vi "Autonomous Independent.vi"() -> ()   [LabVIEW 2013]
doc: "This VI is called when autonomous begins, and will automatically be terminated when autonomous ends. You can carry out timed or sensor driven robot movement independently without needing to return to the caller."
uses:
  Robot Global Data.vi
  <vilib>/Rock Robotics/WPI/RobotDrive/WPI_RobotDriveGetSetRefNum.vi
  <vilib>/Rock Robotics/WPI/RobotDrive/WPI_RobotDriveArcadeDrive_Standard(NoSaturation).vi
  <vilib>/Rock Robotics/WPI/Joystick/WPI_JoystickGetSetRefNum.vi
panel:
  out "Current Movement, for debugging":T1 {"Y Joystick Value" scale=1.0..-1.0; "X Joystick Value" scale=-1.0..1.0}
  in  "Array of robot movements":T2(array[cluster])=[{"X Joystick Value"=0.0, "Y Joystick Value"=0.0, "Delay (sec)"=0.7, "Movement Name"="Lift Arm V", "Joystick Button 1"=FALSE, "Joystick Button 2"=TRUE, "Joystick Button 3"=FALSE, "Joystick Button 4"=FALSE, "Joystick Button 5"=FALSE, "Joystick Button 6"=FALSE, "Joystick Button 7"=FALSE, "Joystick Button 8"=FALSE, "Joystick Button 9"=FALSE, "Joystick Button 10"=FALSE, "Joystick Button 11"=FALSE, "Joystick Button 12"=FALSE}, {"X Joystick Value"=0.0, "Y Joystick Value"=0.0, "Delay (sec)"=0.5, "Movement Name"="Throw Arm V", "Joystick Button 1"=TRUE, "Joystick Button 2"=FALSE, "Joystick Button 3"=FALSE, "Joystick Button 4"=FALSE, "Joystick Button 5"=TRUE, "Joystick Button 6"=FALSE, "Joystick Button 7"=FALSE, "Joystick Button 8"=FALSE, "Joystick Button 9"=FALSE, "Joystick Button 10"=FALSE, "Joystick Button 11"=FALSE, "Joystick Button 12"=FALSE}, {"X Joystick Value"=-0.45, "Y Joystick Value"=-0.75, "Delay (sec)"=3.0, "Movement Name"="Drive Fwd", "Joystick Button 1"=FALSE, "Joystick Button 2"=FALSE, "Joystick Button 3"=FALSE, "Joystick Button 4"=FALSE, "Joystick Button 5"=FALSE, "Joystick Button 6"=FALSE, "Joystick Button 7"=FALSE, "Joystick Button 8"=FALSE, "Joystick Button 9"=FALSE, "Joystick Button 10"=FALSE, "Joystick Button 11"=FALSE, "Joystick Button 12"=FALSE}, {"X Joystick Value"=0.0, "Y Joystick Value"=0.0, "Delay (sec)"=0.5, "Movement Name"="Throw Arm ^", "Joystick Button 1"=TRUE, "Joystick Button 2"=FALSE, "Joystick Button 3"=FALSE, "Joystick Button 4"=FALSE, "Joystick Button 5"=TRUE, "Joystick Button 6"=FALSE, "Joystick Button 7"=FALSE, "Joystick Button 8"=FALSE, "Joystick Button 9"=FALSE, "Joystick Button 10"=FALSE, "Joystick Button 11"=FALSE, "Joystick Button 12"=FALSE}, {"X Joystick Value"=0.0, "Y Joystick Value"=0.0, "Delay (sec)"=1.0, "Movement Name"="Finish", "Joystick Button 1"=FALSE, "Joystick Button 2"=FALSE, "Joystick Button 3"=FALSE, "Joystick Button 4"=FALSE, "Joystick Button 5"=FALSE, "Joystick Button 6"=FALSE, "Joystick Button 7"=FALSE, "Joystick Button 8"=FALSE, "Joystick Button 9"=FALSE, "Joystick Button 10"=FALSE, "Joystick Button 11"=FALSE, "Joystick Button 12"=FALSE}, {"X Joystick Value"=0.0, "Y Joystick Value"=0.0, "Delay (sec)"=0.0, "Movement Name"="", "Joystick Button 1"=FALSE, "Joystick Button 2"=FALSE, "Joystick Button 3"=FALSE, "Joystick Button 4"=FALSE, "Joystick Button 5"=FALSE, "Joystick Button 6"=FALSE, "Joystick Button 7"=FALSE, "Joystick Button 8"=FALSE, "Joystick Button 9"=FALSE, "Joystick Button 10"=FALSE, "Joystick Button 11"=FALSE, "Joystick Button 12"=FALSE}, {"X Joystick Value"=0.0, "Y Joystick Value"=0.0, "Delay (sec)"=0.0, "Movement Name"="", "Joystick Button 1"=FALSE, "Joystick Button 2"=FALSE, "Joystick Button 3"=FALSE, "Joystick Button 4"=FALSE, "Joystick Button 5"=FALSE, "Joystick Button 6"=FALSE, "Joystick Button 7"=FALSE, "Joystick Button 8"=FALSE, "Joystick Button 9"=FALSE, "Joystick Button 10"=FALSE, "Joystick Button 11"=FALSE, "Joystick Button 12"=FALSE}, {"X Joystick Value"=0.0, "Y Joystick Value"=0.0, "Delay (sec)"=0.0, "Movement Name"="", "Joystick Button 1"=FALSE, "Joystick Button 2"=FALSE, "Joystick Button 3"=FALSE, "Joystick Button 4"=FALSE, "Joystick Button 5"=FALSE, "Joystick Button 6"=FALSE, "Joystick Button 7"=FALSE, "Joystick Button 8"=FALSE, "Joystick Button 9"=FALSE, "Joystick Button 10"=FALSE, "Joystick Button 11"=FALSE, "Joystick Button 12"=FALSE}] {"Y Joystick Value" scale=1.0..-1.0; "X Joystick Value" scale=-1.0..1.0}
  # "Be sure to right-click on the ARRAY object (not the individual elements) and choose Data Operations>>Make Current Value default if you want to save the array values with the VI"
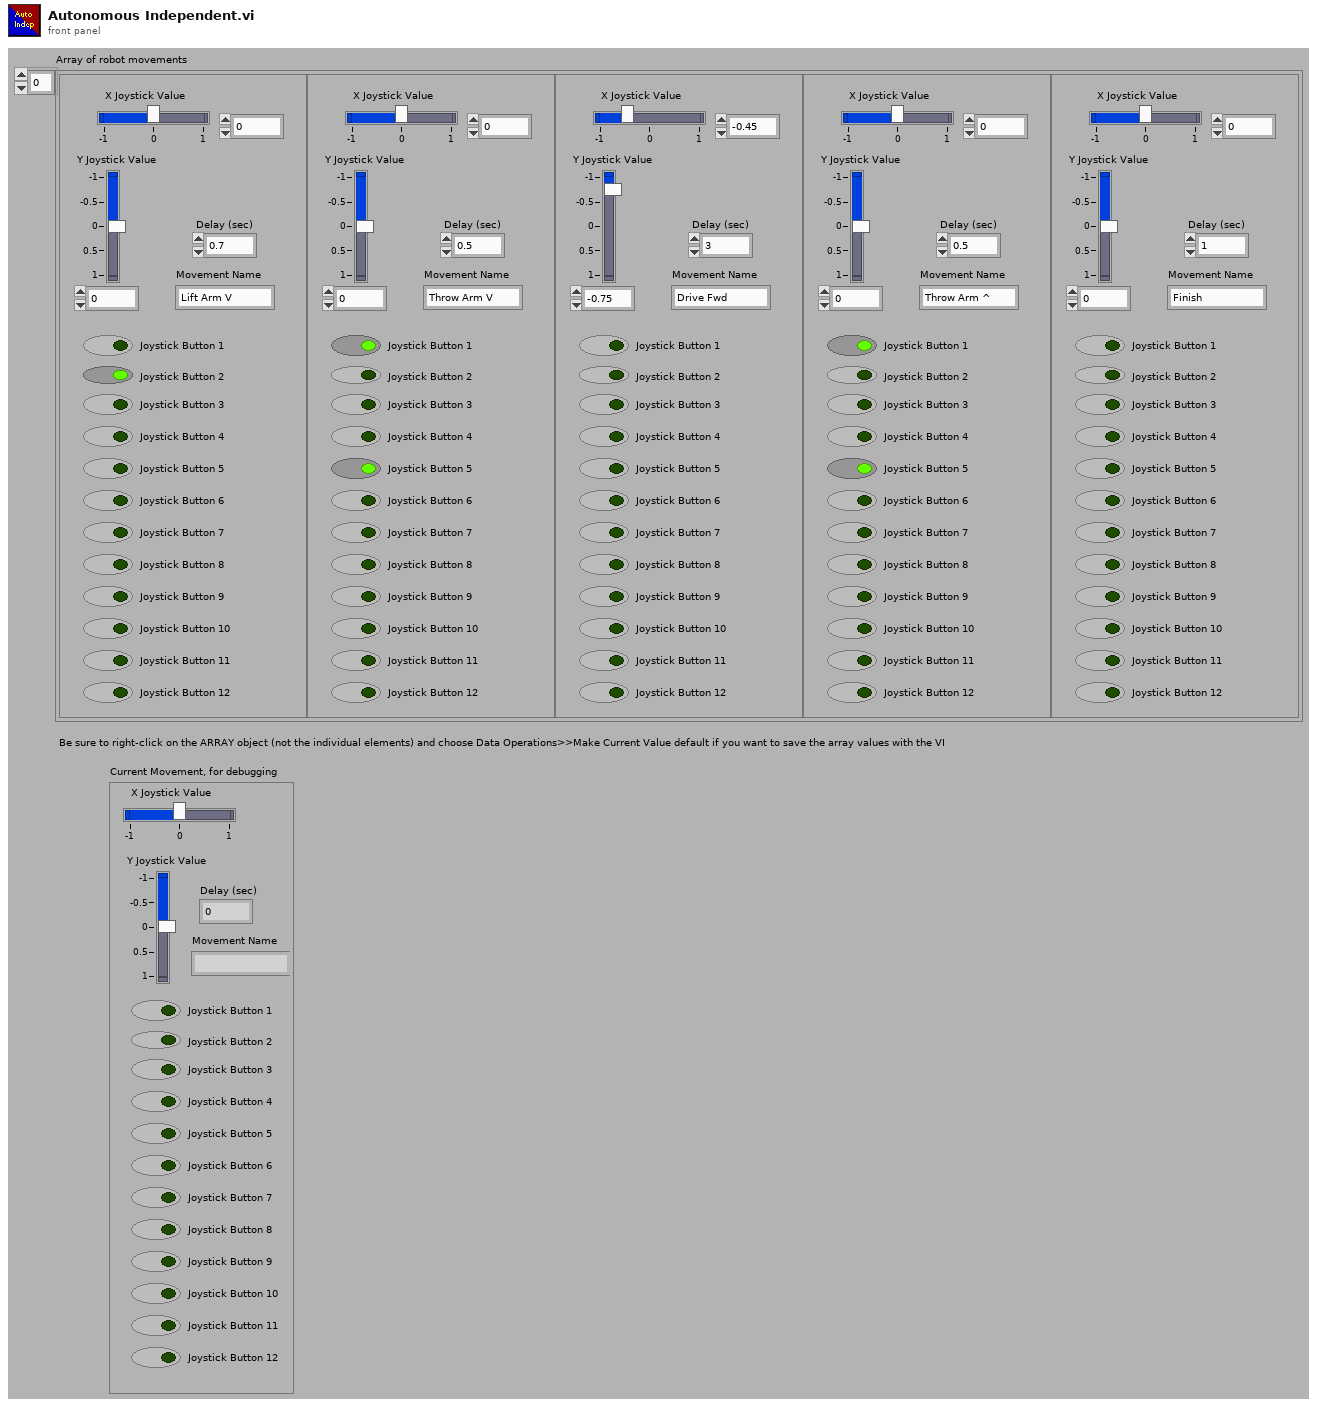
[diagram p1: front panel]
types:
  T1 = cluster{"X Joystick Value":dbl, "Y Joystick Value":dbl, "Delay (sec)":dbl, "Movement Name":string, "Joystick Button 1":bool, "Joystick Button 2":bool, "Joystick Button 3":bool, "Joystick Button 4":bool, "Joystick Button 5":bool, "Joystick Button 6":bool, "Joystick Button 7":bool, "Joystick Button 8":bool, "Joystick Button 9":bool, "Joystick Button 10":bool, "Joystick Button 11":bool, "Joystick Button 12":bool}
  T2 = cluster{"X Joystick Value":dbl, "Y Joystick Value":dbl, "Delay (sec)":dbl, "Movement Name":string, "Joystick Button 1":bool, "Joystick Button 2":bool, "Joystick Button 3":bool, "Joystick Button 4":bool, "Joystick Button 5":bool, "Joystick Button 6":bool, "Joystick Button 7":bool, "Joystick Button 8":bool, "Joystick Button 9":bool, "Joystick Button 10":bool, "Joystick Button 11":bool, "Joystick Button 12":bool}[]
  T3 = typedef "WPI_JoystickDevRef.ctl" = cluster{"Device":T4}
  T4 = typedef "WPI_JoystickDeviceEnum.ctl" = enum16{"USB 1", "USB 2", "USB 3", "USB 4", "Kinect 1", "Kinect 2"}
  T5 = cluster{"axis 1 (x)":dbl, "axis 2 (y)":dbl, "axis 3 (throttle)":dbl, "axis 4":dbl, "axis 5":dbl, "axis 6":dbl}
  T6 = typedef "WPI_RobotDriveDevRef.ctl" = cluster{"DevStatus":errorcluster, "Motors[]":T7[], "Square Inputs":bool, "Max Output":dbl, "Isochronous":bool}
  T7 = typedef "WPI_MotorControlDeviceRef.ctl" = cluster{"DeviceStatus":errorcluster, "Type":enum16{"PWM", "CAN"}, "PWM":cluster{"Digital Module":T8, "PWM Channel":T9, "DeadBand":T10}, "CAN":cluster{"Device Number":u8, "Control Mode":T11, "Semaphore":T12, "Max Vout":dbl}, "Invert":bool, "TransformRef":T13, "InvTransformRef":T13}
  T8 = typedef "FPGA_TypedefDigitalModule.ctl" = enum16{"Digital Module 1", "Digital Module 2"}
  T9 = typedef "FPGA_DIOPWMChannel.ctl" = enum8{"PWM 1", "PWM 2", "PWM 3", "PWM 4", "PWM 5", "PWM 6", "PWM 7", "PWM 8", "PWM 9", "PWM 10", "Invalid"}
  T10 = typedef "WPI_PWMDeadband.ctl" = cluster{"Name":string, "maxPositivePwm":i32, "minPositivePwm":i32, "centerPwm":i32, "maxNegativePwm":i32, "minNegativePwm":i32, "angularRange":u16}
  T11 = typedef "WPI_CANJaguar_ControlMode.ctl" = enum8{"Percent VBus", "Current", "Speed", "Position", "Voltage"}
  T12 = typedef "Semaphore RefNum" = refnum<k1>
  T13 = typedef "WPI_PWMTransform_ConPane.ctl" = refnum<vi>
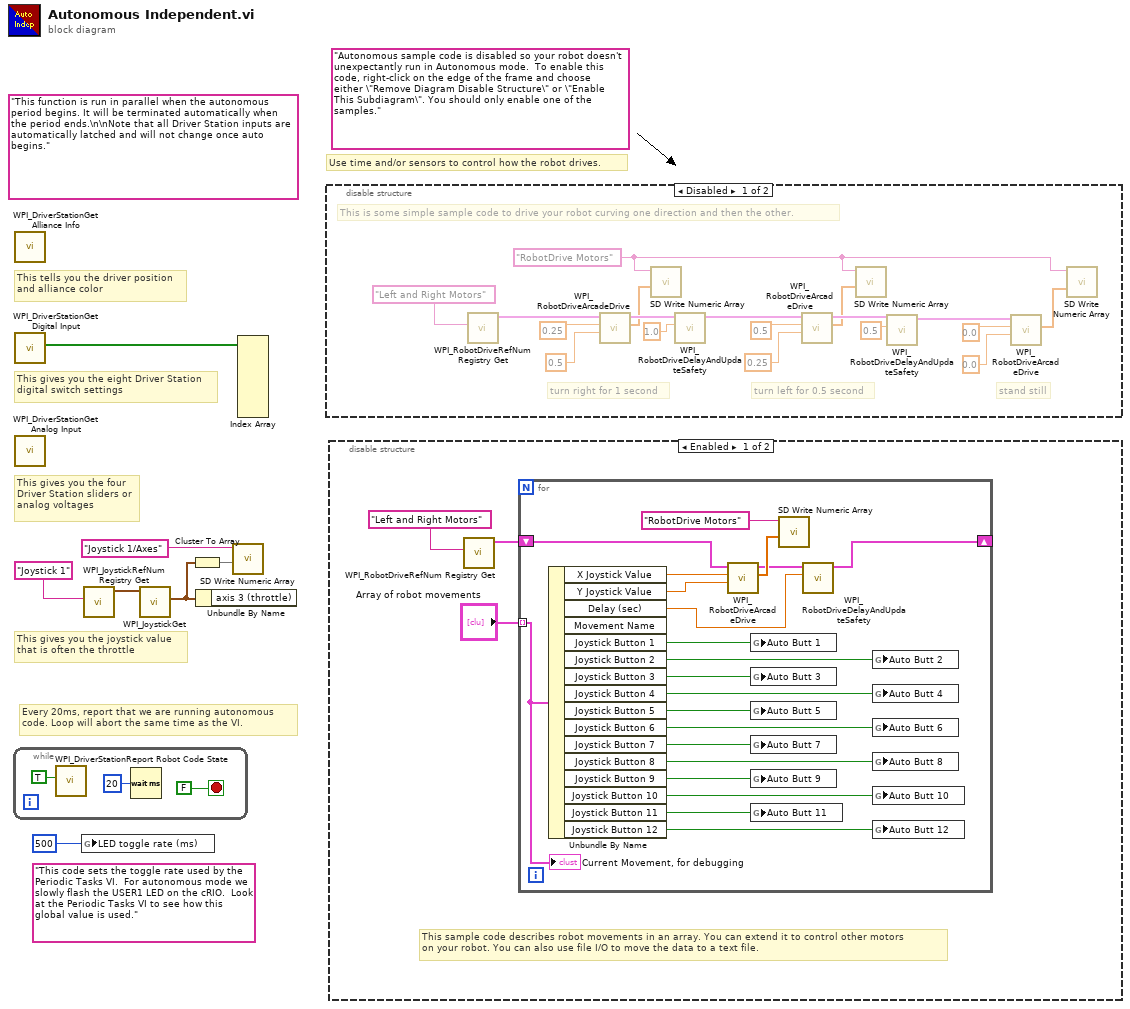
[diagram p0: block diagram]
diagram:
  (unwired) "This code sets the toggle rate used by the Periodic Tasks VI.  For autonomous mode we slowly flash the USER1 LED on the cRIO.  Look at the Periodic Tasks VI to see how this global value is used."
  (unwired) "Autonomous sample code is disabled so your robot doesn't unexpectantly run in Autonomous mode.  To enable this code, right-click on the edge of the frame and choose either \"Remove Diagram Disable Structure\" or \"Enable This Subdiagram\". You should only enable one of the samples."
  (unwired) "This function is run in parallel when the autonomous period begins. It will be terminated automatically when the period ends.\n\nNote that all Driver Station inputs are automatically latched and will not change once auto begins."
  # "Every 20ms, report that we are running autonomous\ncode. Loop will abort the same time as the VI."
  # "This gives you the joystick value\nthat is often the throttle"
  # "Use time and/or sensors to control how the robot drives."
  # "This tells you the driver position\nand alliance color"
  # "This gives you the eight Driver Station\ndigital switch settings"
  # "This gives you the four\nDriver Station sliders or\nanalog voltages"
  n1 = while {
    stop <- FALSE stop-if-true
    n2 = call <vilib>:"WPI_DriverStationReport Robot Code State.vi"("Autonomous"=TRUE) -> ()  [unwired: 10 in, 1 out]
    n3 = Wait (ms)(milliseconds to wait=u32 20) -> ()  [unwired: 1 out]
  }
  n4 = call <vilib>:"WPI_DriverStationGet Alliance Info.vi"() -> ()  [unwired: 12 out]
  n5 = call <vilib>:"WPI_DriverStationGet Digital Input.vi"() -> ("Driver Station Digital Input (1-8)"=w7:bool[])  [unwired: 11 out]
  n6 = call <vilib>:"WPI_DriverStationGet Analog Input.vi"() -> ()  [unwired: 12 out]
  n7 = global write "Robot Global Data.vi" "LED toggle rate (ms)"(u32 500 ("LED ms toggle rate")) -> ()
  n8 = call <vilib>:"WPI_JoystickRefNum Registry Get.vi"("refnum name"="Joystick 1") -> ("JoystickDevRef"=w5:T3)  [unwired: 1 in, 9 out]
  n9 = call <vilib>:"WPI_JoystickGet.vi"("JoystickDevRef"=w5) -> ("Axes"=w2:T5)  [unwired: 1 in, 5 out]
  n10 = Cluster To Array(cluster=w2) -> (array=w3:dbl[])
  n11 = Unbundle By Name(w2) -> ()  [unwired: 1 out]
  n12 = call <vilib>:"SD Write Numeric Array.vi"("Numeric Array"=w3, "Name"="Joystick 1/Axes") -> ()  [unwired: 8 in, 2 out]
  n13 = Index Array(array=w7) -> ()  [unwired: 8 in, 8 out]
  n14 = disable-structure shown="Disabled" {
    frame Disabled {
      w11 = "RobotDrive Motors" ("Name")
      # "This is some simple sample code to drive your robot curving one direction and then the other."
      # "stand still"
      # "turn left for 0.5 second"
      # "turn right for 1 second"
      n15 = call <vilib>:"WPI_RobotDriveRefNum Registry Get.vi"("refnum name"="Left and Right Motors") -> ("RobotDriveDevRef"=w15:T6)  [unwired: 1 in, 9 out]
      n16 = call-poly <vilib>:"WPI_RobotDriveArcadeDrive.vi"("Y axis value"=0.5 ("X axis value"), "X axis value"=0.25, "RobotDriveDevRef"=w15) -> ("Motor Values"=w14:dbl[], "RobotDriveDevRef"=w22:T6)  [unwired: 1 in, 6 out]
      n17 = call <vilib>:"SD Write Numeric Array.vi"("Numeric Array"=w14, "Name"=w11) -> ()  [unwired: 8 in, 2 out]
      n18 = call <vilib>:"WPI_RobotDriveDelayAndUpdateSafety.vi"("Delay (s)"=1.0, "RobotDriveDevRef"=w22) -> ("RobotDriveDevRef 2"=w21:T6)  [unwired: 8 in, 1 out]
      n19 = call-poly <vilib>:"WPI_RobotDriveArcadeDrive.vi"("Y axis value"=0.25 ("X axis value"), "X axis value"=0.5, "RobotDriveDevRef"=w21) -> ("Motor Values"=w13:dbl[], "RobotDriveDevRef"=w20:T6)  [unwired: 1 in, 6 out]
      n20 = call <vilib>:"SD Write Numeric Array.vi"("Numeric Array"=w13, "Name"=w11) -> ()  [unwired: 8 in, 2 out]
      n21 = call <vilib>:"WPI_RobotDriveDelayAndUpdateSafety.vi"("Delay (s)"=0.5, "RobotDriveDevRef"=w20) -> ("RobotDriveDevRef 2"=w19:T6)  [unwired: 8 in, 1 out]
      n22 = call-poly <vilib>:"WPI_RobotDriveArcadeDrive.vi"("Y axis value"=0.0 ("X axis value"), "X axis value"=0.0, "RobotDriveDevRef"=w19) -> ("Motor Values"=w12:dbl[])  [unwired: 1 in, 7 out]
      n23 = call <vilib>:"SD Write Numeric Array.vi"("Numeric Array"=w12, "Name"=w11) -> ()  [unwired: 8 in, 2 out]
    }
    frame Enabled {
    }
  }
  n24 = disable-structure shown="Enabled" {
    frame Enabled {
      # "This sample code describes robot movements in an array. You can extend it to control other motors\non your robot. You can also use file I/O to move the data to a text file."
      n25 = call <vilib>:"WPI_RobotDriveRefNum Registry Get.vi"("refnum name"="Left and Right Motors") -> ("RobotDriveDevRef"=w30:T6)  [unwired: 1 in, 9 out]
      n26 = for {
        shift-right: [w48] -> _
        shift-left: w30 -> [w49]
        tunnel: "Array of robot movements" -> [w44] mode=indexing
        n27 = Unbundle By Name(w44) -> ("X Joystick Value"=w47:dbl, "Y Joystick Value"=w46:dbl, "Delay (sec)"=w45:dbl, "Joystick Button 1"=w43:bool, "Joystick Button 2"=w42:bool, "Joystick Button 3"=w41:bool, "Joystick Button 4"=w40:bool, "Joystick Button 5"=w39:bool, "Joystick Button 6"=w38:bool, "Joystick Button 7"=w37:bool, "Joystick Button 8"=w36:bool, "Joystick Button 9"=w35:bool, "Joystick Button 10"=w34:bool, "Joystick Button 11"=w33:bool, "Joystick Button 12"=w32:bool)  [unwired: 1 out]
        n28 = call-poly <vilib>:"WPI_RobotDriveArcadeDrive.vi"("Y axis value"=w46, "X axis value"=w47, "RobotDriveDevRef"=w49) -> ("Motor Values"=w51:dbl[], "RobotDriveDevRef"=w50:T6)  [unwired: 1 in, 6 out]
        n29 = global write "Robot Global Data.vi" "Auto Butt 1"(w43) -> ()
        n30 = global write "Robot Global Data.vi" "Auto Butt 3"(w41) -> ()
        n31 = global write "Robot Global Data.vi" "Auto Butt 5"(w39) -> ()
        n32 = global write "Robot Global Data.vi" "Auto Butt 7"(w37) -> ()
        n33 = global write "Robot Global Data.vi" "Auto Butt 9"(w35) -> ()
        n34 = global write "Robot Global Data.vi" "Auto Butt 11"(w33) -> ()
        n35 = call <vilib>:"SD Write Numeric Array.vi"("Numeric Array"=w51, "Name"="RobotDrive Motors") -> ()  [unwired: 8 in, 2 out]
        n36 = call <vilib>:"WPI_RobotDriveDelayAndUpdateSafety.vi"("Delay (s)"=w45, "RobotDriveDevRef"=w50) -> ("RobotDriveDevRef 2"=w48:T6)  [unwired: 8 in, 1 out]
        n37 = global write "Robot Global Data.vi" "Auto Butt 2"(w42) -> ()
        n38 = global write "Robot Global Data.vi" "Auto Butt 4"(w40) -> ()
        n39 = global write "Robot Global Data.vi" "Auto Butt 6"(w38) -> ()
        n40 = global write "Robot Global Data.vi" "Auto Butt 8"(w36) -> ()
        n41 = global write "Robot Global Data.vi" "Auto Butt 10"(w34) -> ()
        n42 = global write "Robot Global Data.vi" "Auto Butt 12"(w32) -> ()
        "Current Movement, for debugging" <- w44
      }
    }
    frame Disabled {
    }
  }
